vi "niFpga wdp fft 4-wire wrapper 16spc.vi"(0 "real data in":fxp<+/-,8,1>[](array[numeric])=[0.0, 0.0, 0.0, 0.0, 0.0, 0.0, 0.0, 0.0, 0.0, 0.0, 0.0, 0.0, 0.0, 0.0, 0.0, 0.0], 1 "reset":bool, 5 "imaginary data in":fxp<+/-,8,1>[](array[numeric])=[0.0, 0.0, 0.0, 0.0, 0.0, 0.0, 0.0, 0.0, 0.0, 0.0, 0.0, 0.0, 0.0, 0.0, 0.0, 0.0], 9 "input valid":bool, 12 "ready for output":bool) -> (3 "data indices":u16[](array[numeric]), 4 "real data out":fxp<+/-,19,12>[](array[numeric]), 6 "imaginary data out":fxp<+/-,19,12>[](array[numeric]), 10 "output valid":bool, 14 "ready for input":bool)   [LabVIEW 2017]
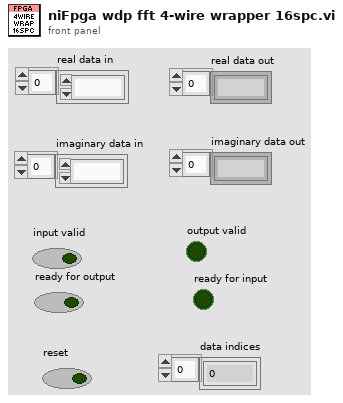
[diagram p1: front panel]
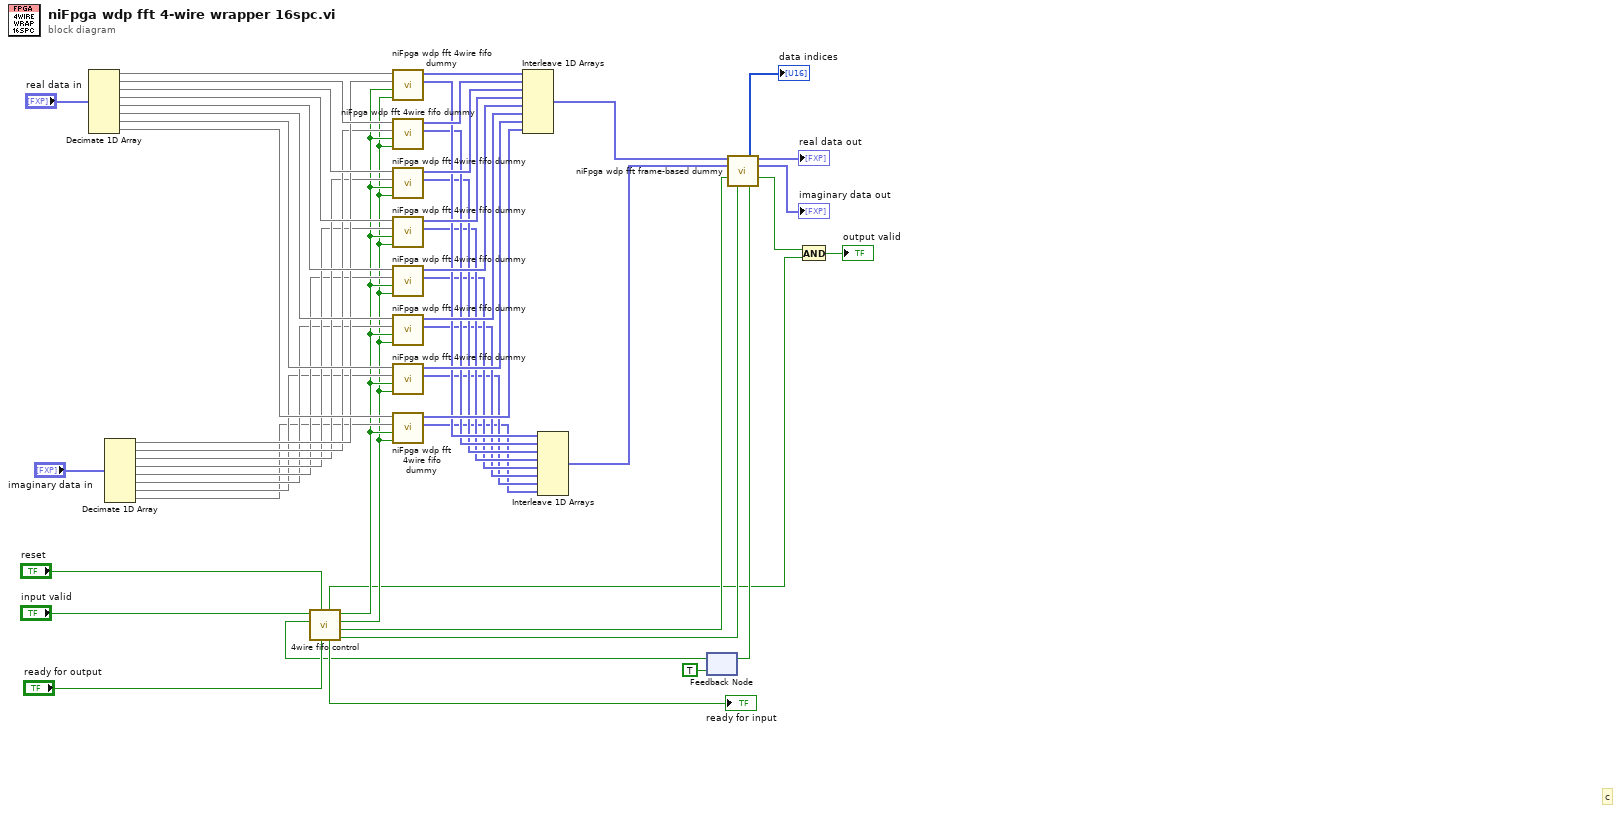
[diagram p0: block diagram]
diagram:
  # "c"
  n1 = Decimate 1D Array("real data in") -> (w45:fxp<+/-,8,1>[], w44:fxp<+/-,8,1>[], w43:fxp<+/-,8,1>[], w42:fxp<+/-,8,1>[], w41:fxp<+/-,8,1>[], w40:fxp<+/-,8,1>[], w39:fxp<+/-,8,1>[], w38:fxp<+/-,8,1>[])
  n2 = Decimate 1D Array("imaginary data in") -> (w36:fxp<+/-,8,1>[], w35:fxp<+/-,8,1>[], w34:fxp<+/-,8,1>[], w33:fxp<+/-,8,1>[], w32:fxp<+/-,8,1>[], w31:fxp<+/-,8,1>[], w30:fxp<+/-,8,1>[], w29:fxp<+/-,8,1>[])
  n3 = feedback #1(TRUE ("ready for frame")) -> (w1:bool)
  n4 = call "4wire fifo control"("ready for output"="ready for output", "reset"="reset", "ready for frame"=w1, "input valid"="input valid") -> ("enable"=w10:bool, "frame start"=w9:bool, "read?"=w7:bool, "write?"=w8:bool, "ready for input"=→"ready for input":bool, "not in reset?"=w6:bool)  [unwired: 2 in]
  n5 = call <vilib>:"niFpga wdp fft 4wire fifo dummy.vi"("read?"=w7, "write?"=w8, "data in im"=w36, "data in re"=w45) -> ("data out im"=w19:fxp<+/-,8,1>[], "data out re"=w28:fxp<+/-,8,1>[])  [unwired: 6 in]
  n6 = call <vilib>:"niFpga wdp fft 4wire fifo dummy.vi"("read?"=w7, "write?"=w8, "data in im"=w35, "data in re"=w44) -> ("data out im"=w18:fxp<+/-,8,1>[], "data out re"=w27:fxp<+/-,8,1>[])  [unwired: 6 in]
  n7 = call <vilib>:"niFpga wdp fft 4wire fifo dummy.vi"("read?"=w7, "write?"=w8, "data in im"=w34, "data in re"=w43) -> ("data out im"=w17:fxp<+/-,8,1>[], "data out re"=w26:fxp<+/-,8,1>[])  [unwired: 6 in]
  n8 = call <vilib>:"niFpga wdp fft 4wire fifo dummy.vi"("read?"=w7, "write?"=w8, "data in im"=w33, "data in re"=w42) -> ("data out im"=w16:fxp<+/-,8,1>[], "data out re"=w25:fxp<+/-,8,1>[])  [unwired: 6 in]
  n9 = call <vilib>:"niFpga wdp fft 4wire fifo dummy.vi"("read?"=w7, "write?"=w8, "data in im"=w32, "data in re"=w41) -> ("data out im"=w15:fxp<+/-,8,1>[], "data out re"=w24:fxp<+/-,8,1>[])  [unwired: 6 in]
  n10 = call <vilib>:"niFpga wdp fft 4wire fifo dummy.vi"("read?"=w7, "write?"=w8, "data in im"=w31, "data in re"=w40) -> ("data out im"=w14:fxp<+/-,8,1>[], "data out re"=w23:fxp<+/-,8,1>[])  [unwired: 6 in]
  n11 = call <vilib>:"niFpga wdp fft 4wire fifo dummy.vi"("read?"=w7, "write?"=w8, "data in im"=w30, "data in re"=w39) -> ("data out im"=w13:fxp<+/-,8,1>[], "data out re"=w22:fxp<+/-,8,1>[])  [unwired: 6 in]
  n12 = call <vilib>:"niFpga wdp fft 4wire fifo dummy.vi"("read?"=w7, "write?"=w8, "data in im"=w29, "data in re"=w38) -> ("data out im"=w12:fxp<+/-,8,1>[], "data out re"=w21:fxp<+/-,8,1>[])  [unwired: 6 in]
  n13 = Interleave 1D Arrays(w28, w27, w26, w25, w24, w23, w22, w21) -> (w20:fxp<+/-,8,1>[])
  n14 = Interleave 1D Arrays(w19, w18, w17, w16, w15, w14, w13, w12) -> (w11:fxp<+/-,8,1>[])
  n15 = call <vilib>:"niFpga wdp fft frame-based dummy.vi"("real data in"=w20, "imaginary data in"=w11, "input frame start"=w9, "enable"=w10) -> ("data indices"=→"data indices":u16[], "real data out"=→"real data out":fxp<+/-,19,12>[], "imaginary data out"=→"imaginary data out":fxp<+/-,19,12>[], "output valid"=w50:bool, "ready for frame"=w48:bool)  [unwired: 6 in, 1 out]
  n16 = feedback-in #1(w48) -> ()
  n17 = And(x=w50, y=w6) -> (x .and. y?=→"output valid":bool)
